vi "LWXPS_PositionerCorrectorPIDDualFFVoltageGet.vi"(0 "XPS Reference IN":refnum<k24>, 2 "Positioner Name":string, 7 "LabVIEW error IN":errorcluster) -> (10 "XPS Reference OUT":refnum<k24>, 11 "LabVIEW error OUT":errorcluster, 12 "Returned error code":i32, 13 "XPS Error String":string, 14 "Closed Loop Status":bool, 15 "Friction":dbl, 16 "Proportional gain":dbl, 17 "Feed Forward Acceleration":dbl, 18 "Integral gain":dbl, 19 "Feed forward velocity":dbl, 20 "Derivative gain":dbl, 21 "Integral saturation value":dbl, 22 "Integration time":dbl, 23 "Derivative filter cut off frequency":dbl, 24 "Proportional gain multiplier":dbl, 25 "Integral gain multiplier":dbl, 26 "Derivative gain multiplier":dbl, 27 "Form coefficient":dbl)   [LabVIEW 2014]
uses:
  D:/XPSQ8_LabView_Library/Development/Source/Dll/Newport.XPS.CommandInterface.dll
  Dll/Newport.XPS.CommandInterface.dll
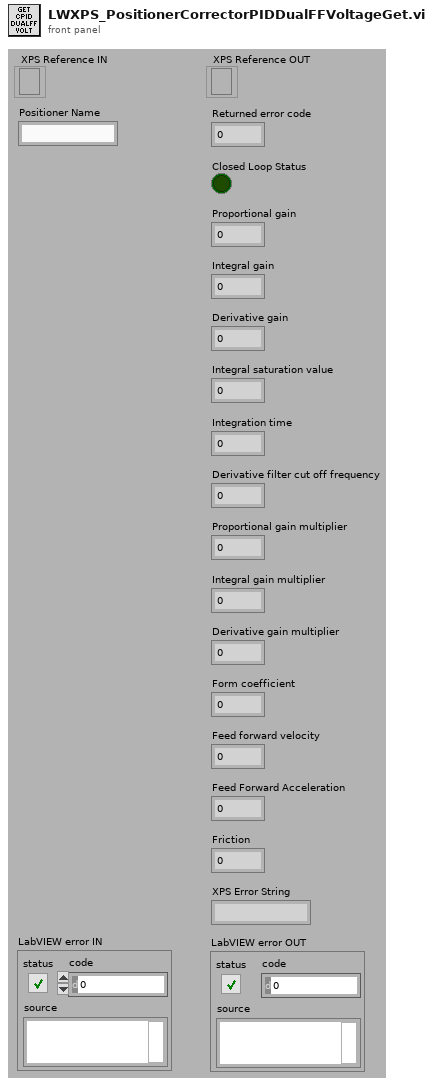
[diagram p1: front panel]
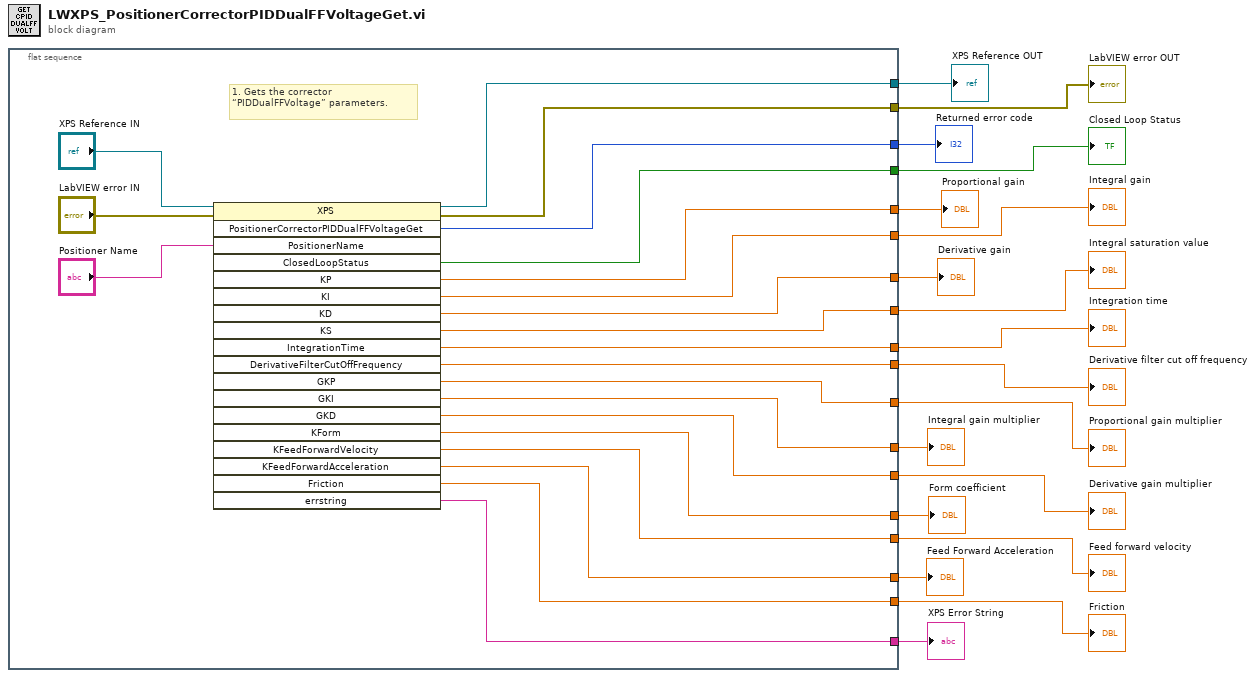
[diagram p0: block diagram]
diagram:
  n1 = flat-sequence {
    tunnel: [w37] -> w10
    tunnel: [w30] -> w18
    tunnel: [w38] -> w17
    tunnel: [w34] -> w16
    tunnel: [w33] -> w2
    tunnel: [w31] -> w15
    tunnel: [w32] -> w14
    tunnel: [w25] -> w13
    tunnel: [w29] -> w11
    tunnel: [w28] -> w12
    tunnel: [w27] -> w1
    tunnel: [w26] -> w5
    tunnel: [w24] -> w9
    tunnel: [w23] -> w8
    tunnel: [w22] -> w7
    tunnel: [w21] -> w3
    tunnel: [w20] -> w6
    tunnel: [w19] -> w4
    frame #0 {
      # "1. Gets the corrector “PIDDualFFVoltage” parameters."
      n2 = invoke class="XPS" method="PositionerCorrectorPIDDualFFVoltageGet"(reference="XPS Reference IN", error in="LabVIEW error IN", "PositionerName"="Positioner Name") -> (reference out=w37:refnum<k24>, error out=w30:errorcluster, "PositionerCorrectorPIDDualFFVoltageGet"=w38:i32, "ClosedLoopStatus"=w29:bool, "KP"=w34:dbl, "KI"=w33:dbl, "KD"=w31:dbl, "KS"=w32:dbl, "IntegrationTime"=w25:dbl, "DerivativeFilterCutOffFrequency"=w28:dbl, "GKP"=w27:dbl, "GKI"=w26:dbl, "GKD"=w24:dbl, "KForm"=w23:dbl, "KFeedForwardVelocity"=w22:dbl, "KFeedForwardAcceleration"=w21:dbl, "Friction"=w20:dbl, "errstring"=w19:string)  [unwired: 16 in, 1 out]
    }
  }
  "XPS Error String" <- w4
  "XPS Reference OUT" <- w10
  "LabVIEW error OUT" <- w18
  "Returned error code" <- w17
  "Proportional gain" <- w16
  "Integral gain" <- w2
  "Derivative gain" <- w15
  "Integral saturation value" <- w14
  "Integration time" <- w13
  "Derivative filter cut off frequency" <- w12
  "Proportional gain multiplier" <- w1
  "Closed Loop Status" <- w11
  "Derivative gain multiplier" <- w9
  "Form coefficient" <- w8
  "Feed forward velocity" <- w7
  "Feed Forward Acceleration" <- w3
  "Friction" <- w6
  "Integral gain multiplier" <- w5
